vi "DecodeEvents.vi"(8 "error in":errorcluster, 9 "array":u8[](array[numeric]), 10 "Key":i32=5) -> (0 "error out":errorcluster, 2 "array w/ subset deleted out":u8[](array[numeric]), 3 "Vector Flags":cluster{"id":dbl, "flag":bool}[](array[cluster]))   [LabVIEW 2017]
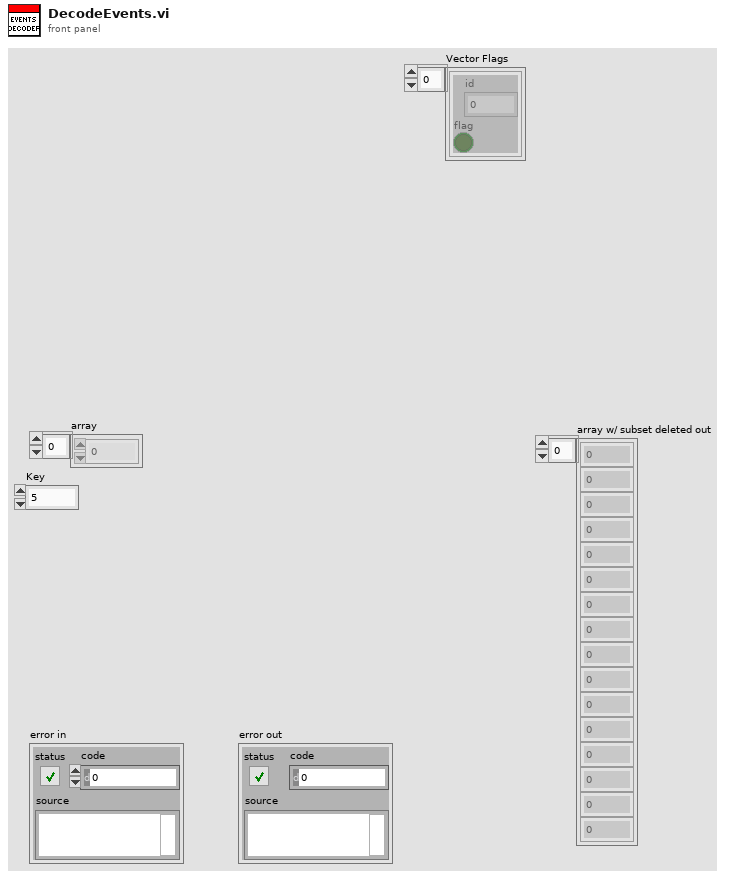
[diagram p1: front panel]
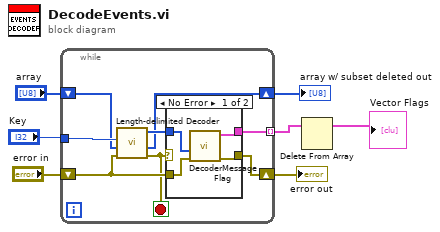
[diagram p0: block diagram]
diagram:
  n1 = while {
    shift-right: [w12] -> w5
    shift-left: "array" -> [w8]
    tunnel: [w15] -> w4 mode=indexing
    shift-right: [w14] -> w7
    shift-left: "error in" -> [w11]
    tunnel: "Key" -> [w9]
    stop <- w10 stop-if-true
    n2 = call "Length-delimited Decoder.vi"("error in (no error)"=w11, "Array"=w8, "Key"=w9) -> ("error out"=w10:errorcluster, "array w/ subset deleted"=w12:u8[], "Length-delimited"=w13:u8[])  [unwired: 5 in, 1 out]
    n3 = case shown="No Error" w10 {
      tunnel: [w16 _] -> w15
      tunnel: [w17 w20] -> w14
      tunnel: w13 -> [w19 _]
      tunnel: w11 -> [w18 w20]
      frame No Error {
        n4 = call "DecoderMessageFlag.vi"("error in"=w18, "Array"=w19) -> ("error IO"=w17:errorcluster, "flags"=w16:cluster{"id":dbl, "flag":bool})  [unwired: 7 in, 1 out]
      }
      frame Error {
      }
    }
  }
  "error out" <- w7
  "array w/ subset deleted out" <- w5
  n5 = Delete From Array(array=w4) -> (array with subset deleted=→"Vector Flags":cluster{"id":dbl, "flag":bool}[])  [unwired: 2 in, 1 out]
